vi "Main VERSION 1.0.vi"() -> ()   [LabVIEW 2017]
uses:
  <vilib>/addons/_Advanced Signal Processing/NI_AdvSigProcWA.lvlib
  <vilib>/addons/_Advanced Signal Processing/NI_AdvSigProcTSA.lvlib
  <vilib>/addons/Control Design/_Model Construction/NI_LinSys_Model Creation.lvlib
  <vilib>/addons/Control Design/_Model Conversions/NI_CD_Continuous and Discrete.lvlib
  <vilib>/addons/Control Design/_Model Construction/Data Typedefs.llb/CD DtoC Conversion Method.ctl
  <vilib>/addons/Control Design/_Model Construction/NI_LinSys_Data Typedefs.lvlib
  <vilib>/Analysis/NI_AALBase.lvlib
  Data.ctl
  <vilib>/Math Plots/3D Math Plots/3D Surface/3D Surface Datatype/3D Surface Datatype.lvclass
  <vilib>/addons/Control Design/_Dynamic Analysis/NI_CD_Dynamic Analysis.lvlib
  <vilib>/platform/TimedLoop/XDataNode/XDataNode.xnode
  <vilib>/Platform/TimedLoop/XDataNode/nitl_modes.ctl
  <vilib>/Platform/TimedLoop/XDataNode/XDNodeRunTimeDep.lvlib
  <vilib>/Platform/TimedLoop/XDataNode/wakeup.ctl
  <vilib>/Platform/TimedLoop/XDataNode/timing_clust.ctl
  <vilib>/addons/Control Design/_Model Construction/Model Creation.llb/Model Creation SubVI/cd_Create Transfer Function Model.vi
  <vilib>/addons/Control Design/_Model Conversions/NI_CD_Model Type.lvlib
  <vilib>/Analysis/NI_AALPro.lvlib
  <vilib>/addons/Control Design/_Time Response Analysis/NI_CD_Time Response.lvlib
  <vilib>/Utility/file.llb/Read Delimited Spreadsheet (DBL).vi
  <vilib>/ptbypt/NI_PtbyPt.lvlib
  <vilib>/Utility/file.llb/Write Delimited Spreadsheet (DBL).vi
  <vilib>/addons/Control Design/_Dynamic Analysis/Dynamic Analysis.llb/Dynamic Analysis subVI/cd_Damping Ratio and Natural Frequency (State-Space).vi
  <vilib>/addons/Control Design/_Time Response Analysis/Time Response.llb/Time Response subVI/cd_Linear Simulation (Transfer Function).vi
  <vilib>/addons/Control Design/_Model Conversions/Continuous and Discrete.llb/Continuous and Discrete SubVI/cd_Convert Discrete to Continuous (TF).vi
  <vilib>/addons/Time Series Analysis/Modeling and Prediction.llb/TSA ARMA Modeling (Waveform).vi
  <vilib>/addons/Control Design/_Dynamic Analysis/Dynamic Analysis.llb/Dynamic Analysis subVI/cd_Damping Ratio and Natural Frequency (Transfer Function).vi
  <vilib>/addons/Control Design/_Model Conversions/Model Type.llb/Model Conversion SubVI/cd_Convert Transfer Function to State-Space Model.vi
  <vilib>/Analysis/3filter.llb/IIR Filter (DBL).vi
  <vilib>/addons/Wavelet Analysis/application.llb/WA Detrend (Waveform).vi
  <vilib>/addons/Time Series Analysis/Correlation and Spectral Analysis.llb/TSA ARMA Spectrum (Waveform).vi
  <vilib>/Math Plots/3D Math Plots/3D Surface/3D Surface Datatype/Public/Plot Helper (Vector).vi
  State.ctl
  <vilib>/Math Plots/3D Math Plots/3D Surface/3D Surface XCtrl/3D Surface.xctl
panel:
  out "Poles":cdb[](array[numeric]) format="%.2f"
  out "Damping Ratios":dbl[](array[numeric]) format="%.2f"
  out "Natural Frequencies":dbl[](array[numeric]) format="%.2f"
  out "subarray 2":dbl[](array[numeric])
  out "AR coeff test 2":dbl[](array[numeric])=[1.0, -3.469, 4.669, -2.879, 0.6897]
  out "subarray":dbl[][](array[numeric])
  in  "Tab Control 2":enum32{"Data", "Preprocessed data"}(tab)
  out "Real-time data":waveform(dbl)(graph)={"t0"=timestamp(3467964116.0127993 s since 1904-01-01), "dt"=0.02, "Y"=array[30000 elements]}
  out "Preprocessed data":waveform(dbl)(graph)={"t0"=timestamp(3467964116.0127993 s since 1904-01-01), "dt"=0.2, "Y"=array[3000 elements]}
  in  "Tab Control":T1(tab)=enum."Options"
  out "Critical Damping [%]":dbl=11.530156484123282
  out "Critical Frequency [Hz]":dbl=1.626086044993813
  out "Estimated complex plane":cluster{dbl[], dbl[]}(graph)={[-1.1780360817698377, -0.5023745738423925, -1.9397187258807729], [10.148858009104277, 3.227170083530164, 12.249765461704891]}
  out "Damping ratio evolution":dbl[][](graph)=[[11.530156484123282, 8.701215529283058, 2.189395909955882, 2.4614029943222535, 5.193514233637378, 4.3692184421257805, 4.91283055168465, 4.380817107946644, 2.1306948942275286, 8.227924724815844, 2.674410475393449, 9.21941081019913]]
  in  "Number of critical modes":i32=1
  in  "Length of Spectra [s]":dbl=12.0
  out "Spectrogram":refnum<class "3D Plot Datatype.lvclass">[](xcontrol)
  in  "dB Scale":bool=TRUE
  out "Spectrum":cluster{"f0":dbl, "df":dbl, "S(f)":dbl[]}(graph)={"f0"=0.0, "df"=0.0048828125, "S(f)"=[53.04783210228587, 56.63653445699592, 58.023891931913106, 59.67116404097662, 61.284054847341054, 62.76981524500722, 64.11687043737376, 65.33794997742491, 66.45015373901528, 67.46886875000477, 68.40631100060692, 69.27151565501251, 70.07073014946974, 70.80788585589455, 71.48506608411563, 72.10296533438401, 72.66135194305483, 73.15953947791074, 73.59685537036363, 73.97307660858725, 74.28878941943108, 74.54562919953614, 74.74637114057295, 74.89486760408374, 74.99585665068564, 75.05468730953243, 75.0770149019896, 75.06851380977426, 75.03464026528596, 74.98046048345269, 74.91054484865359, 74.82891934483663, 74.73906102646188, 74.64392380160663, 74.54598253767928, 74.44728617051356, 74.34951322777977, 74.25402551961022, 74.1619175504306, 74.0740604811893, 73.99114030974818, 73.9136904467079, 73.84211914252114, 73.7767323478459, 73.71775262048499, 73.66533466900506, 73.61957807164293, 73.5805376459866, 73.54823188003344, 73.52264977404724, 73.50375638784266, 73.49149734072392, 73.4858024713342, 73.48658883165905, 73.49376316265318, 73.50722397761325, 73.52686336266768, 73.55256859076123, 73.58422363541801, 73.62171066243388, 73.66491157037783, 73.71370964298946, 73.76799136641728, 73.82764844926844, 73.89258006024016, 73.96269526207116, 74.03791556557854, 74.1181774458125, 74.20343454441851, 74.29365911777792, 74.38884207004048, 74.48899062945569, 74.59412239354747, 74.70425411613539, 74.81938331104598, 74.93946063995493, 75.06435135111367, 75.19378503485144, 75.32729498078686, 75.46415167436817, 75.6032993266386, 75.74330901487231, 75.88236539108851, 76.01830367318581, 76.14870760287604, 76.27106668197574, 76.38297473443528, 76.48233722171956, 76.567548282804, 76.63760408035796, 76.69213526024357, 76.73136176637777, 76.75599006111887, 76.76708083903773, 76.76591406961832, 76.75387077046256, 76.73234153456316, 76.70266377607953, 76.6660844104162, 76.62374225963825, 76.57666412087157, 76.5257692499374, 76.47187827374617, 76.41572380516381, 76.35796107933896, 76.29917770086449, 76.23990210798334, 76.18061067647423, 76.1217335591145, 76.06365943561697, 76.00673936964108, 75.95128995956487, 75.89759594482322, 75.8459123998421, 75.79646661853478, 75.74945976672043, 75.70506835869804, 75.66344559760455, 75.62472260666664, 75.58900956937647, 75.55639679030908, 75.52695568412523, 75.50073969773588, 75.4777851692011, 75.45811212635587, 75.4417250281344, 75.42861345190909, 75.41875273072952, 75.41210454504176, 75.40861747421977, 75.40822751400344, 75.41085856667677, 75.41642291151614, 75.42482166367071, 75.43594523019257, 75.44967377239409, 75.46587768405924, 75.48441809525055, 75.50514741151336, 75.52790989815483, 75.55254231893963, 75.57887463796702, 75.606730792646, 75.63592954453935, 75.66628541338444, 75.69760969780361, 75.72971158409061, 75.76239934201378, 75.795481603843, 75.82876871983562, 75.8620741802788, 75.8952160909746, 75.92801868588295, 75.96031385763509, 75.99194268394, 76.02275692567179, 76.05262047079196, 76.0814106973545, 76.10901972876889, 76.13535555532907, 76.16034299778357, 76.18392449140839, 76.20606067257935, 76.22673075411002, 76.2459326804616, 76.26368305914585, 76.28001687001027, 76.29498695938368, 76.30866333104413, 76.32113225044141, 76.33249518238651, 76.34286758537615, 76.35237758776404, 76.36116457208469, 76.36937769399348, 76.37717436156206, 76.38471869915384, 76.3921800179218, 76.399731312252, 76.40754779837235, 76.41580550799458, 76.4246799463977, 76.43434482091358, 76.44497084244557, 76.45672459952794, 76.46976750158741, 76.48425478555691, 76.50033457786182, 76.51814700209086, 76.537823321419, 76.55948510411083, 76.58324340025439, 76.60919791832202, 76.6374361913053, 76.66803272411654, 76.70104811679032, 76.73652816184644, 76.77450291907336, 76.81498577698629, 76.85797251727257, 76.90344040650483, 76.95134734798053, 77.00163113524022, 77.0542088569138, 77.10897650910722, 77.16580887543216, 77.22455973475066, 77.28506245152305, 77.34713099231259, 77.41056139398341, 77.475133684643, 77.54061422858938, 77.6067584336654, 77.67331372673053, 77.74002267438226, 77.80662610573624, 77.87286608565972, 77.93848859279498, 78.00324577763865, 78.06689771036126, 78.12921357240282, 78.18997229504036, 78.24896269622393, 78.30598320836378, 78.36084131989398, 78.41335286956605, 78.46334133381099, 78.51063723532924, 78.55507777800551, 78.59650678285838, 78.63477496585358, 78.66974056458548, 78.70127028997815, 78.72924055336367, 78.75353889979947, 78.77406556576946, 78.79073507334817, 78.80347777292985, 78.8122412518888, 78.81699153604242, 78.81771402347431, 78.81441410508471, 78.807117442166, 78.79586988743347, 78.78073705146184, 78.76180353070973, 78.7391718257197, 78.7129609882886, 78.68330504420013, 78.65035124345292, 78.61425819290841, 78.57519392716361, 78.53333397258037, 78.48885945721293, 78.44195531637583, 78.39280864032669, 78.34160720757664, 78.28853824527842, 78.23378745760364, 78.1775383646809, 78.11997199928643, 78.06126701696634, 78.00160028874863, 77.94114806552857, 77.88008783149982, 77.81860100322533, 77.75687668454131, 77.69511676008476, 77.63354270795473, 77.57240464286238, 77.51199327525148, 77.45265570160778, 77.39481624025024, 77.33900390797915, 77.28588860152158, 77.23632858870927, 77.19143246487005, 77.15263912661203, 77.12181919737093, 77.10139998238675, 77.09451208662946, 77.10514698357909, 77.1382975261337, 77.20002317838411, 77.29733540865345, 77.43774052768978, 77.62823161225614, 77.87354824854364, 78.17371984562733, 78.52135621237176, 78.89977446830142, 79.2834689612792, 79.64200391820367, 79.94678678707898, 80.17810549628706, 80.32909021423254, 80.40498736340558, 80.41896645675713, 80.38714023757896, 80.32483671152525, 80.2447019035565, 80.15623070884602, 80.06607714178779, 79.97864663238913, 79.89669770700486, 79.8218432814422, 79.75492917142036, 79.69630395356339, 79.64600440896002, 79.6038796954954, 79.56967279153454, 79.54307288267267, 79.52374832109005, 79.51136675797247, 79.50560689714834, 79.50616483455582, 79.51275694395522, 79.52512059701962, 79.5430135589285, 79.56621260467892, 79.59451170608011, 79.62772001095674, 79.66565975190154, 79.70816416702898, 79.75507547967509, 79.80624296130985, 79.86152108773445, 79.92076779005671, 79.98384279707365, 80.05060606328794, 80.1209162760194, 80.19462943540331, 80.27159750214368, 80.35166710948391, 80.43467833782597, 80.52046355267608, 80.60884630905795, 80.69964032816455, 80.79264855477103, 80.88766230675424, 80.98446053089533, 81.08280918189732, 81.18246074412212, 81.28315391780771, 81.38461349329644, 81.48655043790035, 81.58866222022453, 81.69063339583282, 81.7921364758338, 81.8928330960746, 81.99237549899337, 82.09040833272722, 82.18657076287359, 82.28049888163618, 82.37182838750634, 82.46019749706196, 82.54525004031949, 82.6266386843919, 82.70402822988488, 82.77709893456618, 82.84554984510027, 82.90910216821055, 82.96750279929881, 83.0205282664879, 83.06798956633493, 83.10973870024924, 83.14567821839111, 83.17577580604392, 83.20008697857843, 83.21879033153864, 83.23224144991188, 83.24105310440208, 83.24620954319899, 83.24921870324471, 83.25229252868525, 83.25851394982814, 83.27189246791492, 83.29713858822798, 83.33895686091842, 83.40078581729284, 83.48329369452597, 83.5834075564926, 83.6946918626584, 83.80914630314666, 83.9194939800654, 84.02078048103141, 84.11077450135917, 84.18945935657379, 84.25819390539944, 84.31896225289465, 84.37386809960977, 84.42486082458214, 84.47362219262848, 84.52154491008937, 84.56975518463469, 84.6191513946612, 84.67044469704172, 84.72419543129335, 84.7808433678376, 84.84073180065857, 84.90412625530703, 84.9712287814767, 85.0421887491838, 85.11711092933817, 85.1960614866747, 85.27907237543178, 85.366144514999, 85.4572500341974, 85.55233380573867, 85.65131444275491, 85.75408489337823, 85.86051274404058, 85.97044032496017, 86.08368470022344, 86.2000376184273, 86.31926549679474, 86.44110951099279, 86.56528586366412, 86.69148630607677, 86.81937898845217, 86.94860971456819, 87.07880367424393, 87.20956772236228, 87.3404932642739, 87.47115979393969, 87.60113911239554, 87.73000022976, 87.85731492419461, 87.98266389667822, 88.10564342253977, 88.22587236147383, 88.3429993499442, 88.4567099666591, 88.56673363657677, 88.67285002492687, 88.77489467267074, 88.8727636403219, 88.96641695838639, 89.05588072856739, 89.1412477774557, 89.22267682950323, 89.30039023358225, 89.37467034199577, 89.44585469740042, 89.51433022763241, 89.58052667814718, 89.6449095255229, 89.70797261362961, 89.77023073836328, 89.83221238000688, 89.8944527475736, 89.95748726030781, 90.02184555101928, 90.08804603676572, 90.15659106659064, 90.22796262489769, 90.30261854328616, 90.380989153439, 90.46347429869138, 90.55044061170233, 90.64221895956518, 90.73910195507645, 90.84134143317605, 90.94914579438051, 91.062677122183, 91.18204798899406, 91.30731787566103, 91.43848914369735, 91.57550251820746, 91.71823206462797, 91.8664796756997, 92.01996912871296, 92.17833982935551, 92.34114042963648, 92.50782259498837, 92.67773530013969, 92.85012015289084, 93.02410837428519, 93.19872019281603, 93.37286752304267, 93.54536087204167, 93.71492142038328, 93.88019912304051, 94.03979743538294, 94.19230486438343, 94.33633296933988, 94.47055971554589, 94.5937762851988, 94.70493468147838, 94.80319286424029, 94.88795387440493, 94.9588955525746, 95.01598807987202, 95.05949761483718, 95.0899756234817, 95.1082348876195, 95.1153144006739, 95.1124362317316, 95.10095785179813, 95.08232336383243, 95.05801663917848, 95.02951866998893, 94.99827064726611, 94.96564349614025, 94.93291393519425, 94.90124662329674, 94.87168162629092, 94.84512626132259, 94.82235032847149, 94.80398378321688, 94.79051600716397, 94.78229597263946, 91.76923279427284]}
  out "AR Coeff":dbl[](array[numeric])=[1.0, 0.2597816046489246, 0.2169384834121149, -0.679920142435816, -0.14595364680322792, 0.05002853302205009, 0.4579510483015735, 0.33236397122107786, -0.23625030751664058, -0.18717706840003662, -0.2062523669387352, 0.006685880060599296, 0.07110018702253204, 0.058723568346406144, 0.029083213351701387, 0.04124721740773827, 0.05689913231139613, 0.03808009033984788, 0.03677353221719321, 0.025432779832026717, 0.047521341239954946, 0.030318507891188288, 0.0798326201716732, 0.020455322957894737, 0.031484626629290524, -0.006461565839629831]
  out "MA Coeff":dbl[](array[numeric])=[1.0, -0.6848360549660951, 0.6884899387060236, -1.383587023284228, 0.9145041211231907, -0.7466132797884354, 0.988179180636961, -0.5622742582232239, 0.09840748978464724, -0.26486368933416604, -0.03646716818404465]
  out "Picture 9":picture
  out "Picture 8":picture
  out "Picture 7":picture
  out "Picture 6":picture
  out "Picture 5":picture
  out "Picture 4":picture
  out "Picture 3":picture
  out "Picture 2":picture
  out "Picture 1":picture
  out "Std of Damping":dbl[](array[numeric])=[3.167813045881809]
  out "Mean Damping [%]":dbl[](array[numeric])=[5.49924934647624]
  out "Frequency[Hz]":dbl[](array[numeric])=[1.626086044993813, 0.5198061588603065, 1.9739015777045272] format="%.4f"
  out "Damping Ratio [%]":dbl[](array[numeric])=[11.530156484123282, 15.381771713903165, 15.639879258359347] format="%.4f"
  out "Complex Poles":cdb[](array[numeric])=[-1.1780360817698377+10.148858009104277i, -0.5023745738423925+3.227170083530164i, -1.9397187258807729+12.249765461704891i] format="%.4f"
  out "Format":string="a0*z^4+a1*z^3+a2*z^2+a3*z^1+a4"
  out "Format":string="b0*z^3+b1*z^2+b2*z^1+b3"
  in  "MA coeff test":dbl[](array[numeric])=[1.0, -2.175, 1.45, 5.0]
  in  "AR coeff test":dbl[](array[numeric])=[1.0, -3.469, 4.669, -2.879, 0.6897]
  in  "Simulation/PRL":bool=TRUE
  in  "Upper Damping [%]":dbl=20.0
  in  "Lower Damping [%]":dbl
  in  "Upper Frequency [Hz]":dbl=2.0
  in  "Lower Frequency [Hz]":dbl=0.08
  in  "Signal Selection":enum32{"Mag", "Phase", "Analog"}(radio)=enum."Analog"
  in  "Downsampling Ratio":dbl=10.0
  in  "Low-pass Filter [Hz]":dbl=2.5
  in  "Low-pass Filter Order":u32=5
  in  "Detrend Cut-off Frequency":dbl=0.05
  in  "MA Order":i32=10
  in  "Sampling Frequency":dbl=50.0
  in  "AR Order":i32=25
  in  "Parcel Length (Simulation)":i32=30000
  in  "Refresh Rate [s]":i32=10
  in  "Std Threshold":dbl=1.35
  out "Parcel Length (SDK or Simulation)":i32=30000
  out "Simulation":bool=TRUE
  in  "stop":bool
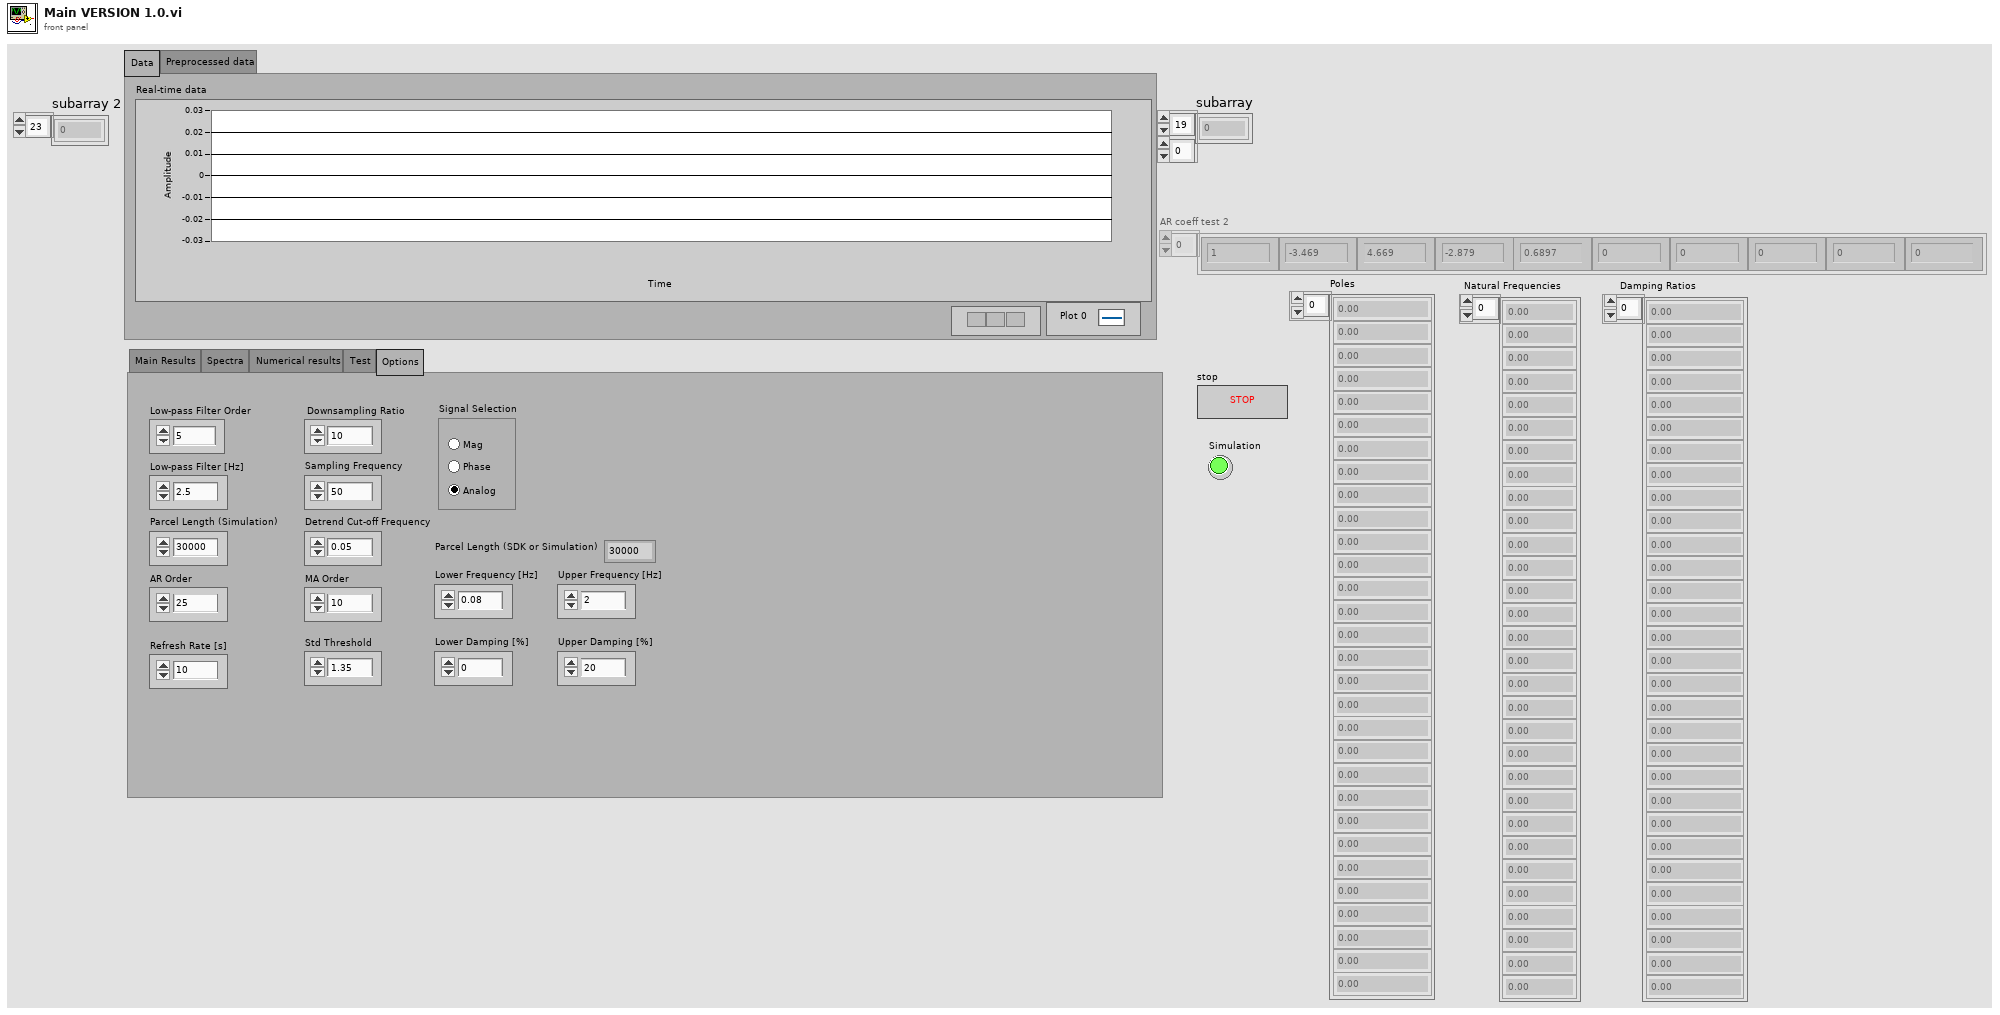
[diagram p1: front panel]
types:
  T1 = enum32{"Main Results", "Spectra", "Numerical results", "Test", "Options"}
  T2 = typedef "State.ctl" = enum16{"Initialize", "Read Real Data", "Read Simulated Data", "Preprocessing", "Compute AR/MA Coeffs", "Get Spectrum"}
  T3 = typedef "Data.ctl" = cluster{"Waveform":waveform(dbl), "Parcel Length":i32, "AR Order":i32, "Sampling Frequency":dbl, "MA Order ":i32}
  T4 = typedef "XDNodeRunTimeDep.lvlib/timing_clust.ctl" = cluster{"Expected End [f-1]":u64, "Actual End [f-1]":u64, "Finished Late? [f-1]":bool, "Expected End [i-1]":u64, "Actual End [i-1]":u64, "Finished Late? [i-1]":bool, "Expected Start [i]":u64, "Actual Start [i]":u64, "Expected Start [f]":u64, "Actual Start [f]":u64, "Source Name":string, "Structure Name":string, "Period":i64, "Deadline":i64, "Offset":i64, "Start":i64, "Priority":i32, "Timeout":i32, "Mode":T5, "Wakeup Reason":T6, "Error":errorcluster, "Source Type":string, "Secondary Source Type":string, "Global End Time":u64, "Global Start Time":u64, "Frame Duration":u64, "Iteration Duration":u64, "Assigned CPU":i32, "I/O Scan Engine Mode":u32}
  T5 = typedef "XDNodeRunTimeDep.lvlib/nitl_modes.ctl" = enum32{"No Change", "Process missed periods, maintain original phase", "Discard missed periods, maintain original phase", "Process missed periods, ignore original phase", "Discard missed periods, ignore original phase"}
  T6 = typedef "XDNodeRunTimeDep.lvlib/wakeup.ctl" = enum32{"Normal", "Aborted", "Asynchronous wakeup", "Timing source error", "Timed loop error", "Timeout"}
  T7 = typedef "State.ctl" = enum16{"Initialize", "Read Real Data", "Read Simulated Data", "Preprocessing", "Compute AR Coeff", "Get Spectrum"}
  T8 = enum8{"Enabled", "Disabled", "Disabled and Grayed Out"}
  T9 = typedef "NI_LinSys_Model Typedefs.lvlib/CD Transfer Function Model (MIMO).ctl" = cluster{"properties":T10, "transfer function(s)":T11[][]}
  T10 = typedef "NI_LinSys_Model Typedefs.lvlib/CD General Elements.ctl" = cluster{"Model name":string, "Input names":string[], "Output names":string[], "Input Delays":dbl[], "Output Delays":dbl[], "Sampling Time":dbl, "Notes":string}
  T11 = typedef "NI_LinSys_Model Typedefs.lvlib/CD Transfer Function Model (SISO).ctl" = cluster{"Numerator":dbl[], "Denominator":dbl[], "delay":dbl}
  T12 = typedef "NI_LinSys_Data Typedefs.lvlib/CD MIMO Time Response Data.ctl" = cluster{"Time":dbl[], "Outputs Data":dbl[][][], "States Data":dbl[][][], "plot type":T13}
  T13 = typedef "NI_LinSys_Data Typedefs.lvlib/CD Plot Types Enum.ctl" = enum16{"bode-magnitude", "bode-phase", "nichols", "nyquist", "singular values", "step", "impulse", "initial", "simulation", "nyquist with separation"}
  T14 = typedef "NI_LinSys_Data Typedefs.lvlib/CD DtoC Conversion Method.ctl" = u16
  T15 = typedef "NI_LinSys_Model Typedefs.lvlib/CD State Space Model (MIMO).ctl" = cluster{"properties":T10, "A":dbl[][], "B":dbl[][], "C":dbl[][], "D":dbl[][], "StateNames":string[], "Transport Delay":dbl[][]}
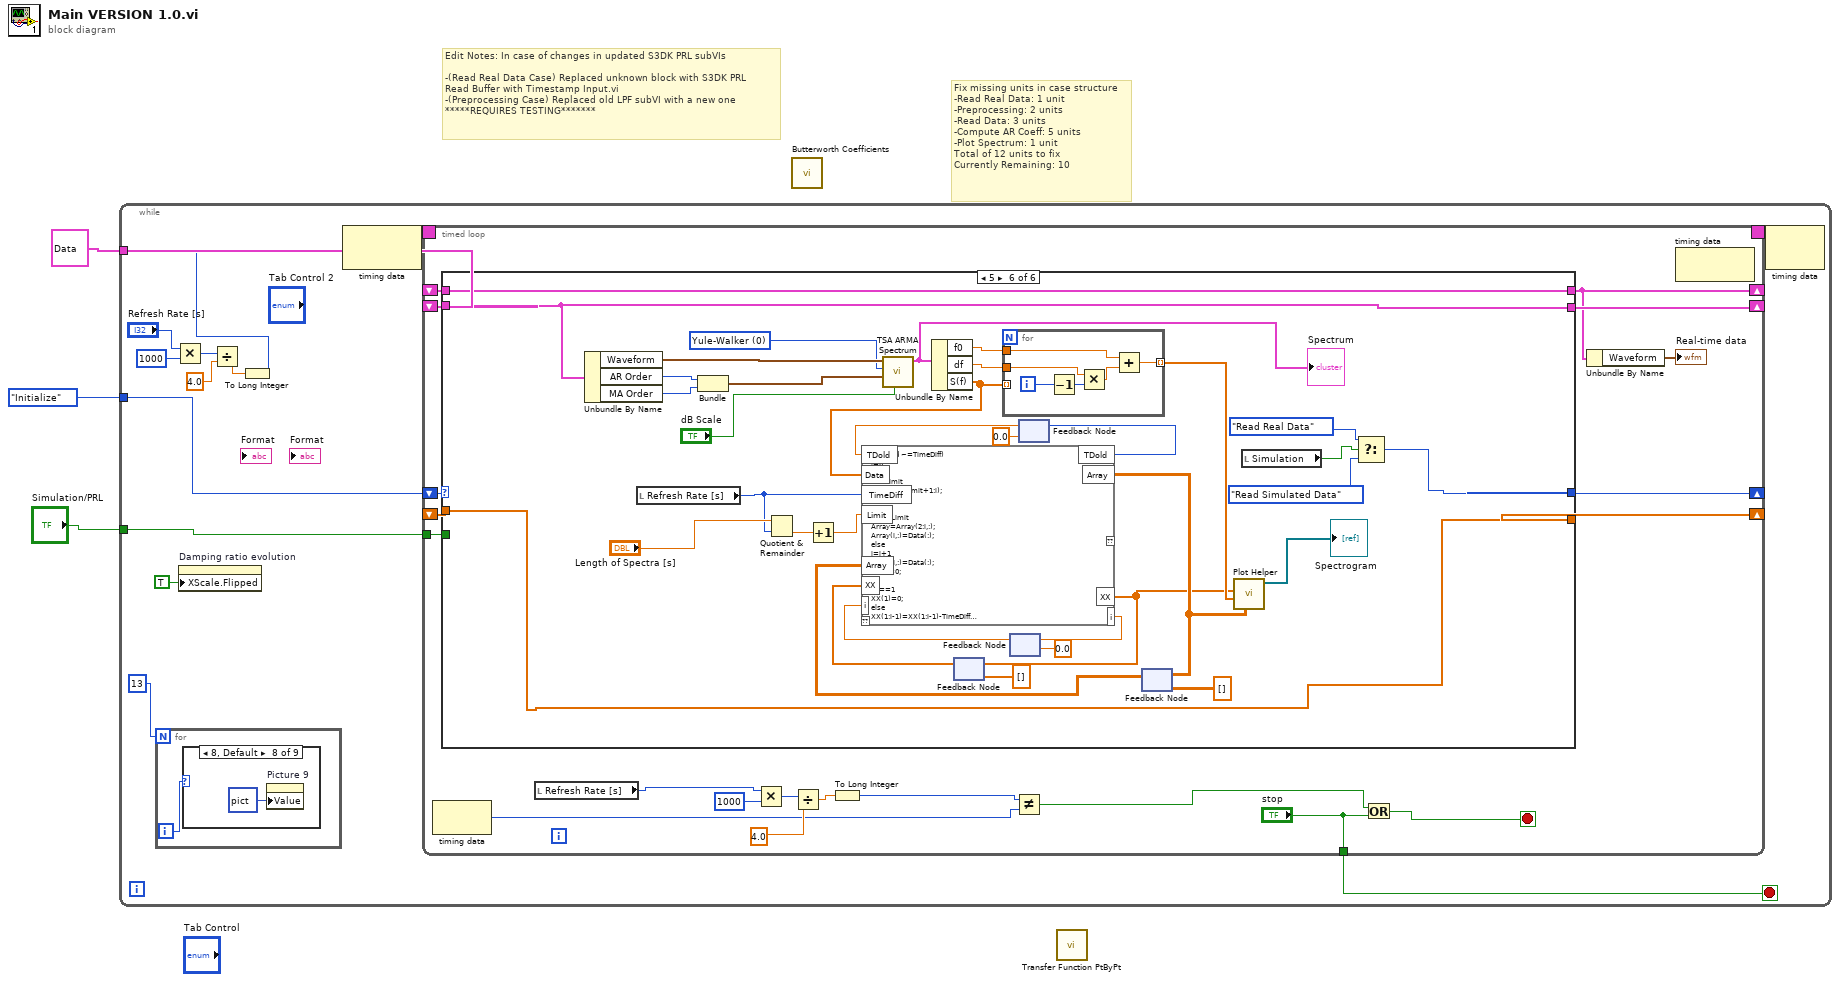
[diagram p0: block diagram]
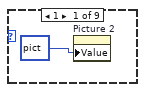
[diagram p2: hidden frame]
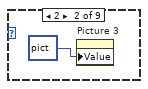
[diagram p3: hidden frame]
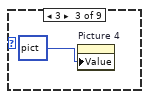
[diagram p4: hidden frame]
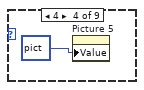
[diagram p5: hidden frame]
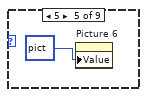
[diagram p6: hidden frame]
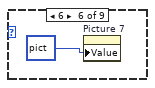
[diagram p7: hidden frame]
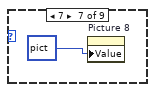
[diagram p8: hidden frame]
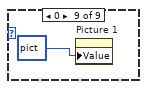
[diagram p9: hidden frame]
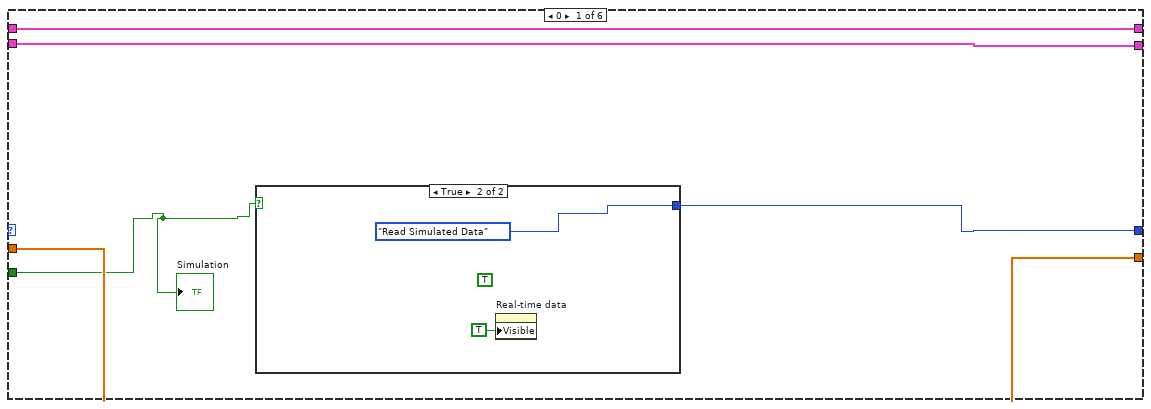
[diagram p10: hidden frame]
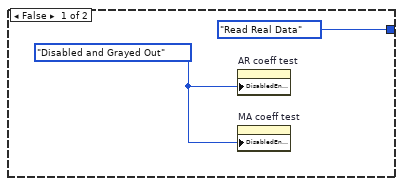
[diagram p11: hidden frame]
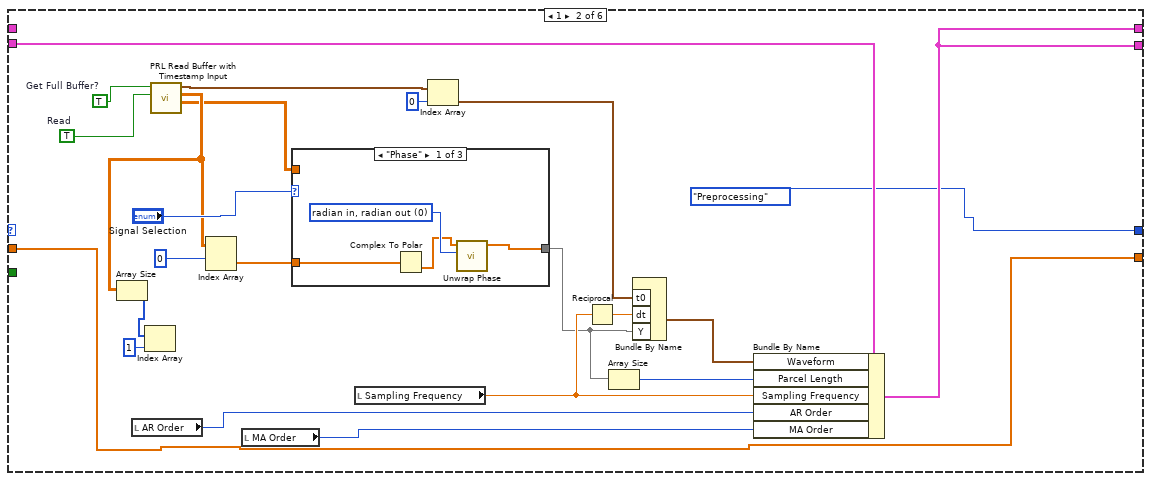
[diagram p12: hidden frame]
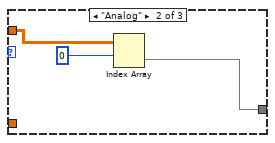
[diagram p13: hidden frame]
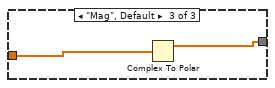
[diagram p14: hidden frame]
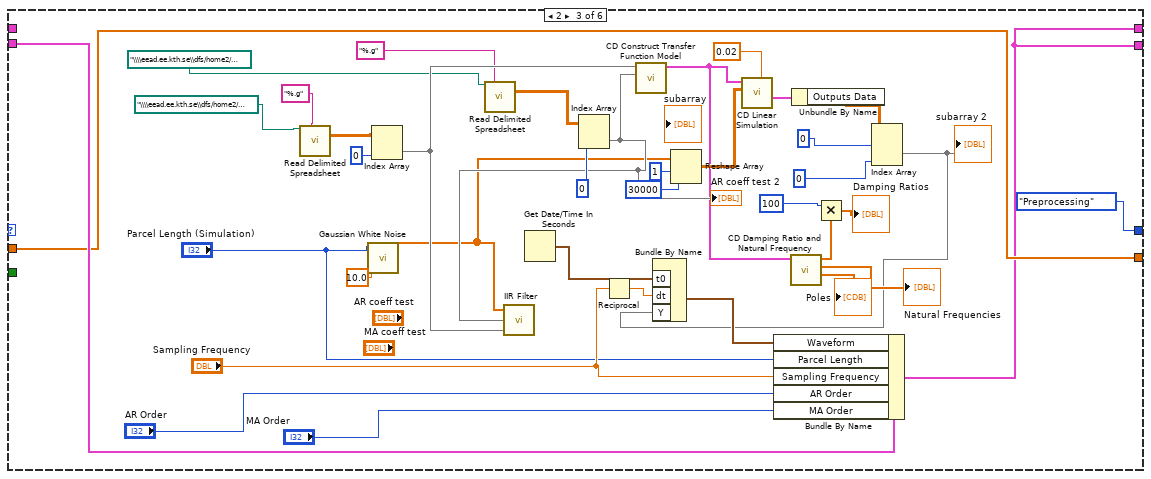
[diagram p15: hidden frame]
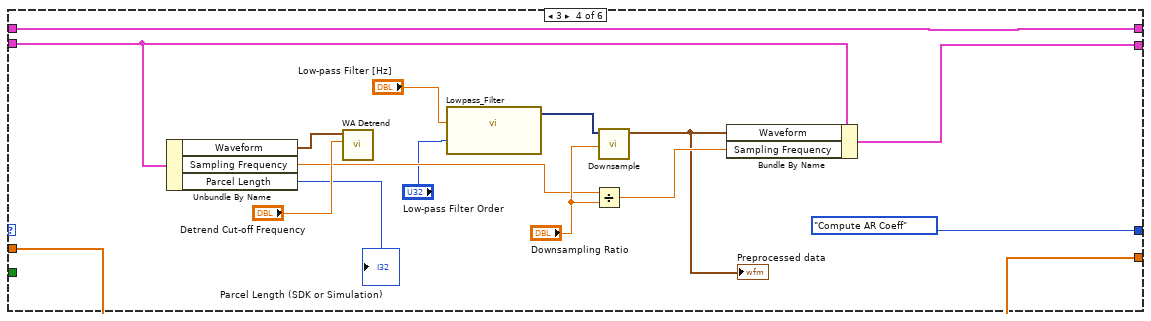
[diagram p16: hidden frame]
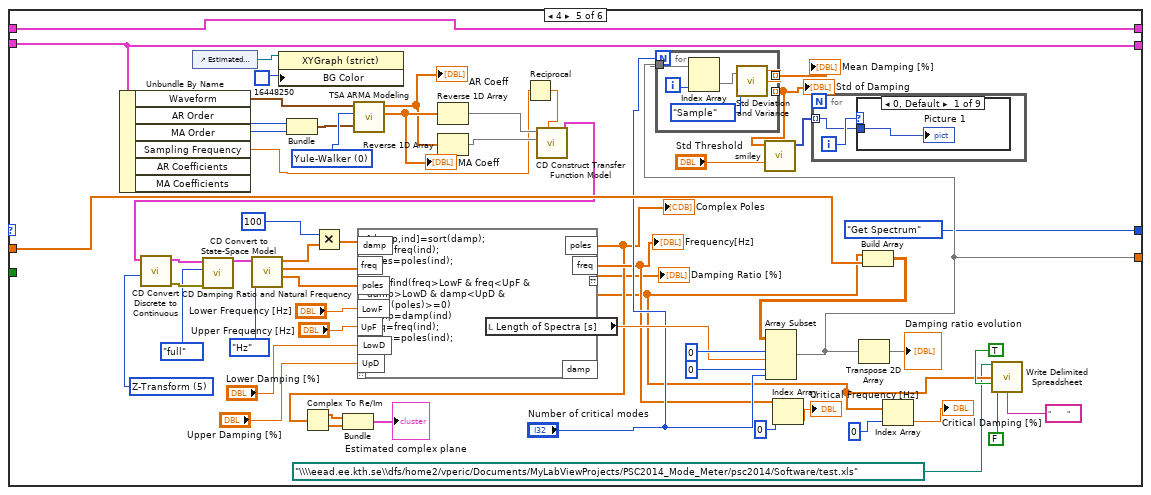
[diagram p17: hidden frame]
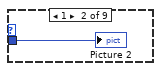
[diagram p18: hidden frame]
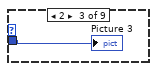
[diagram p19: hidden frame]
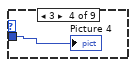
[diagram p20: hidden frame]
diagram:
  # "Edit Notes: In case of changes in updated S3DK PRL subVIs\n\n-(Read Real Data Case) Replaced unknown block with S3DK PRL\nRead Buffer with Timestamp Input.vi  \n-(Preprocessing Case) Replaced old LPF subVI with a new one\n*****REQUIRES TESTING*******"
  # "Fix missing units in case structure\n-Read Real Data: 1 unit\n-Preprocessing: 2 units\n-Read Data: 3 units\n-Compute AR Coeff: 5 units\n-Plot Spectrum: 1 unit\nTotal of 12 units to fix\nCurrently Remaining: 10"
  n1 = while {
    tunnel: State."Initialize" ("Enum") -> [w7]
    tunnel: T3 {"Waveform"={"t0"=timestamp(0 s since 1904-01-01), "dt"=1.0, "Y"=[]}, "Parcel Length"=0, "AR Order"=0, "Sampling Frequency"=0.0, "MA Order "=0} ("Cluster") -> [w15]
    tunnel: "Simulation/PRL" -> [w5]
    stop <- w8 stop-if-true
    n2 = for {
      N: 13 -> [_]
      i -> [w18]
      n3 = case shown="8, Default" w18 {
        frame 1 {
          n4 = property on="Picture 2" class="Pict"("Value"=picture bytes[260130] ("Picture 9")) -> ()  [unwired: 2 in, 2 out]
        }
        frame 2 {
          n5 = property on="Picture 3" class="Pict"("Value"=picture bytes[260130] ("Picture 9")) -> ()  [unwired: 2 in, 2 out]
        }
        frame 3 {
          n6 = property on="Picture 4" class="Pict"("Value"=picture bytes[260130] ("Picture 9")) -> ()  [unwired: 2 in, 2 out]
        }
        frame 4 {
          n7 = property on="Picture 5" class="Pict"("Value"=picture bytes[260130] ("Picture 9")) -> ()  [unwired: 2 in, 2 out]
        }
        frame 5 {
          n8 = property on="Picture 6" class="Pict"("Value"=picture bytes[260130] ("Picture 9")) -> ()  [unwired: 2 in, 2 out]
        }
        frame 6 {
          n9 = property on="Picture 7" class="Pict"("Value"=picture bytes[260130] ("Picture 9")) -> ()  [unwired: 2 in, 2 out]
        }
        frame 7 {
          n10 = property on="Picture 8" class="Pict"("Value"=picture bytes[260130] ("Picture 9")) -> ()  [unwired: 2 in, 2 out]
        }
        frame 8, Default {
          n11 = property on="Picture 9" class="Pict"("Value"=picture bytes[260130] ("Picture 9")) -> ()  [unwired: 2 in, 2 out]
        }
        frame 0 {
          n12 = property on="Picture 1" class="Pict"("Value"=picture bytes[260130] ("Picture 9")) -> ()  [unwired: 2 in, 2 out]
        }
      }
    }
    n13 = Multiply(x="Refresh Rate [s]", y=1000) -> (x*y=w12:i32)
    n14 = property on="Damping ratio evolution" class="WFGraph (strict)"("XScale.Flipped"=TRUE ("X Scale.Flipped")) -> ()  [unwired: 2 in, 2 out]
    n15 = Divide(x=w12, y=4.0) -> (x/y=w10:dbl)
    n16 = To Long Integer(number=w10) -> (32bit integer=w9:i32)
    n17 = node-c288(w9) -> (w17:T4)
    n18 = timed-loop {
      shift-right: [w32] -> _
      shift-left: w15 -> [w46]
      shift-right: [w45] -> _
      shift-left: w7 -> [w47]
      timing: w17 -> [_]
      timing-out: [_] -> w16
      tunnel: ["stop"] -> w8
      shift-right: [w35] -> _
      shift-left: _ -> [w34]
      tunnel: w5 -> [w33]
      shift-right: [w30] -> _
      shift-left: _ -> [w29]
      stop <- w44 stop-if-true
      n19 = node-c288() -> (w28:i64)  [unwired: 1 in]
      n20 = case shown="5" w47 {
        tunnel: w46 -> [w54 w77 w129 w137 w201 w237]
        tunnel: [w54 w68 w121 w144 w201 w237] -> w32
        tunnel: [w55 State."Preprocessing" ("Enum") State."Preprocessing" ("Enum") State."Compute AR Coeff" ("Enum") State."Get Spectrum" ("Enum") w235] -> w45
        tunnel: [w53 w70 w122 w138 w176 w231] -> w35
        tunnel: w34 -> [w53 w70 w122 w138 w189 w231]
        tunnel: w33 -> [w52 _ _ _ _ _]
        tunnel: [w51 w68 w121 w136 w180 w226] -> w30
        tunnel: w29 -> [w51 _ _ w136 w180 w226]
        frame 0 {
          n21 = case shown="True" w52 {
            tunnel: [State."Read Real Data" ("Enum") State."Read Simulated Data" ("Enum")] -> w55
            frame False {
              w57 = T8."Disabled and Grayed Out" ("Disabled")
              n22 = property on="AR coeff test" class="Arr (strict)"("DisabledEnum"=w57) -> ()  [unwired: 2 in, 2 out]
              n23 = property on="MA coeff test" class="Arr (strict)"("DisabledEnum"=w57) -> ()  [unwired: 2 in, 2 out]
            }
            frame True {
              (unwired) TRUE ("Visible")
              n24 = property on="Real-time data" class="WFChart (strict)"("Visible"=TRUE) -> ()  [unwired: 2 in, 2 out]
            }
          }
          "Simulation" <- w52
        }
        frame 1 {
          w64 = TRUE  # Read
          w65 = TRUE  # Get Full Buffer?
          n25 = local read "AR Order"() -> (w80:i32)
          n26 = call <vilib>:"PRL Read Buffer with Timestamp Input.vi"("Get All Signals"=w64, "Get Full Buffer"=w65) -> ("Analog Signals"=w61:sgl[][], "Phasor Signals"=w62:csg[][], "Timestamp"=w63:timestamp[])  [unwired: 3 in, 4 out]
          n27 = Array Size(array=w62) -> (size(s)=w71:i32[])
          n28 = Index Array(array=w71, index=1) -> ()  [unwired: 1 out]
          n29 = Index Array "Index Array"(array=w62, index (row)=0) -> (element=w73:csg[])  [unwired: 1 in]
          n30 = local read "MA Order"() -> (w78:i32)
          n31 = case shown="\"Phase\"" "Signal Selection" {
            tunnel: [w83 w87 w91] -> w66
            tunnel: w73 -> [w86 _ w90]
            tunnel: w61 -> [_ w88 _]
            frame "Phase" {
              w85 = 0 items=["radian in, radian out", "radian in, degree out", "degree in, degree out", "degree in, radian out"] ("phase unit")
              n32 = Complex To Polar(r * e^(i*theta)=w86) -> (theta=w84:sgl[])  [unwired: 1 out]
              n33 = call <vilib>:"Unwrap Phase.vi"("phase unit"=w85, "Phase"=w84) -> ("Unwrapped Phase"=w83:dbl[])  [unwired: 8 in, 1 out]
            }
            frame "Analog" {
              n34 = Index Array(array=w88, index (row)=0) -> (element=w87:sgl[])  [unwired: 1 in]
            }
            frame "Mag", Default {
              n35 = Complex To Polar(r * e^(i*theta)=w90) -> (r=w91:sgl[])  [unwired: 1 out]
            }
          }
          n36 = local read "Sampling Frequency"() -> (w79:dbl)
          n37 = Index Array(array=w63, index=0) -> (element=w75:timestamp)
          n38 = Reciprocal(x=w79) -> (1/x=w82:dbl)
          n39 = Array Size(array=w66) -> (size(s)=w67:i32)
          n40 = Bundle By Name("t0"=w75, "dt"=w82, "Y"=w66) -> (w81:waveform(dbl))  [unwired: 1 in]
          n41 = Bundle By Name(cluster=w77, "Waveform"=w81, "Parcel Length"=w67, "Sampling Frequency"=w79, "AR Order"=w80, "MA Order"=w78) -> (w68:T3)
        }
        frame 2 {
          n42 = call-poly <vilib>:"Read Delimited Spreadsheet.vi"("file path (dialog if empty)"=path "\\\\eead.ee.kth.se\\dfs/home2/vperic/Documents/MyLabViewProjects/PSC2014_Mode_Meter/psc2014/Software/num.txt", "format (%.3f)"="%.g") -> ("all rows"=w97:dbl[][])  [unwired: 8 in, 5 out]
          n43 = call <vilib>:"Gaussian White Noise.vi"("standard deviation"=10.0, "samples"="Parcel Length (Simulation)") -> ("Gaussian noise pattern"=w114:dbl[])  [unwired: 8 in, 1 out]
          n44 = Index Array(array=w97, index (col)=0 ("disabled index (col)")) -> (element=w116:dbl[])  [unwired: 1 in]
          n45 = call-poly <vilib>:"Read Delimited Spreadsheet.vi"("file path (dialog if empty)"=path "\\\\eead.ee.kth.se\\dfs/home2/vperic/Documents/MyLabViewProjects/PSC2014_Mode_Meter/psc2014/Software/den.txt", "format (%.3f)"="%.g") -> ("all rows"=w96:dbl[][])  [unwired: 8 in, 5 out]
          n46 = Get Date/Time In Seconds() -> (seconds since 1Jan1904=w120:timestamp)
          n47 = Index Array(array=w96, index (col)=0 ("disabled index (col)")) -> (element=w115:dbl[])  [unwired: 1 in]
          "AR coeff test 2" <- w115
          n48 = call-poly <vilib>:"IIR Filter.vi"("Forward Coefficients"=w116, "Reverse Coefficients"=w115, "X"=w114) -> ()  [unwired: 1 in, 2 out]
          n49 = Reciprocal(x="Sampling Frequency") -> (1/x=w125:dbl)
          n50 = call-poly <vilib>:"CD Construct Transfer Function Model.vi"("Denominator"=w115, "Numerator"=w116) -> ("Transfer Function Model"=w107:T9)  [unwired: 8 in, 1 out]
          n51 = Reshape Array(w114, 1 ("dimension size"), 30000 ("dimension size")) -> (w113:dbl[][])
          n52 = call-poly <vilib>:"CD Linear Simulation.vi"("Delta t"=0.02, "Inputs"=w113, "Transfer Function Model"=w107) -> ("Simulation Data"=w112:T12)  [unwired: 6 in, 2 out]
          n53 = call-poly <vilib>:"CD Damping Ratio and Natural Frequency.vi"("Transfer Function Model"=w107) -> ("Poles"=→"Poles":cdb[], "Natural Frequencies"=→"Natural Frequencies":dbl[], "Damping Ratios"=w103:dbl[])  [unwired: 7 in, 1 out]
          n54 = Unbundle By Name(w112) -> ("Outputs Data"=w109:dbl[][][])
          n55 = Multiply(x=100 ("length"), y=w103) -> (x*y=→"Damping Ratios":dbl[])
          n56 = Index Array(array=w109, index (dim 0)=0 ("index"), index (dim 2)=0 ("length")) -> (element=w93:dbl[])  [unwired: 1 in]
          "subarray 2" <- w93
          n57 = Bundle By Name("t0"=w120, "dt"=w125, "Y"=w93) -> (w126:waveform(dbl))  [unwired: 1 in]
          n58 = Bundle By Name(cluster=w129, "Waveform"=w126, "Parcel Length"="Parcel Length (Simulation)", "Sampling Frequency"="Sampling Frequency", "AR Order"="AR Order", "MA Order"="MA Order") -> (w121:T3)
        }
        frame 3 {
          n59 = Unbundle By Name(w137) -> ("Waveform"=w132:waveform(dbl), "Sampling Frequency"=w140:dbl, "Parcel Length"=→"Parcel Length (SDK or Simulation)":i32)
          n60 = call-poly <vilib>:"WA Detrend.vi"("threshold frequency"="Detrend Cut-off Frequency", "signal"=w132) -> ()  [unwired: 7 in, 3 out]
          n61 = call "Lowpass_Filter.vi"("Order"="Low-pass Filter Order", "Lower Cut-Off"="Low-pass Filter [Hz]") -> ("Filtered Signal"=w131:dynamicdata)  [unwired: 3 in, 1 out]
          n62 = Divide(x=w140, y="Downsampling Ratio") -> (x/y=w139:dbl)
          n63 = call "Downsample.vi"("Divide by"="Downsampling Ratio", "Waveform in"=w131) -> ("Waveform out"=w135:waveform(dbl))  [unwired: 9 in]
          "Preprocessed data" <- w135
          n64 = Bundle By Name(cluster=w137, "Waveform"=w135, "Sampling Frequency"=w139) -> (w144:T3)
        }
        frame 4 {
          w199 = T14 5 items=["Zero-Order-Hold", "Tustin (Bilinear)", "Prewarp", "Forward", "Backward", "Z-Transform"] ("Method")
          w202 = u16 0 items=["Yule-Walker", "High order AR", "Polynomial"] ("method")
          n65 = Unbundle By Name(w201) -> ("Waveform"=w200:waveform(dbl), "AR Order"=w198:i32, "MA Order"=w197:i32, "Sampling Frequency"=w164:dbl)  [unwired: 2 out]
          n66 = control-ref of="Estimated complex plane"() -> (w192:refnum<vi>)
          n67 = property class="XYGraph (strict)"(reference=w192, "BG Color"=u32 16448250 ("Color Box")) -> ()  [unwired: 1 in, 2 out]
          n68 = Bundle("AR Order"=w198, "MA Order"=w197) -> (w196:cluster{"AR Order":i32, "MA Order ":i32})  [unwired: 1 in]
          n69 = call-poly <vilib>:"TSA ARMA Modeling.vi"("ARMA order"=w196, "method"=w202, "Xt"=w200) -> ("MA coefficients"=w158:dbl[], "AR coefficients"=w157:dbl[])  [unwired: 5 in, 2 out]
          "AR Coeff" <- w157
          "MA Coeff" <- w158
          n70 = Reverse 1D Array(array=w158) -> (reversed array=w172:dbl[])
          n71 = Reverse 1D Array(array=w157) -> (reversed array=w171:dbl[])
          n72 = local read "Length of Spectra [s]"() -> (w183:dbl)
          n73 = Reciprocal(x=w164) -> (1/x=w163:dbl)
          n74 = call-poly <vilib>:"CD Construct Transfer Function Model.vi"("Sampling Time (s)"=w163, "Denominator"=w171, "Numerator"=w172) -> ("Transfer Function Model"=w173:T9)  [unwired: 7 in, 1 out]
          n75 = call-poly <vilib>:"CD Convert Discrete to Continuous.vi"("Method"=w199, "Discrete Transfer Function Model"=w173) -> ("error out"=w162:errorcluster, "Continuous Transfer Function Model"=w151:T9)  [unwired: 8 in]
          n76 = call-poly <vilib>:"CD Convert to State-Space Model.vi"("error in (no error)"=w162, "Realization Type"=enum16{"minimum", "full"}."full", "Transfer Function Model"=w151) -> ("State-Space Model"=w160:T15)  [unwired: 7 in, 1 out]
          n77 = call-poly <vilib>:"CD Damping Ratio and Natural Frequency.vi"("Frequency Unit"=enum16{"Hz", "rad/s"}."Hz", "State-Space Model"=w160) -> ("Poles"=w174:cdb[], "Natural Frequencies"=w165:dbl[], "Damping Ratios"=w184:dbl[])  [unwired: 6 in, 1 out]
          n78 = Multiply(x=100 ("Numeric"), y=w184) -> (x*y=w182:dbl[])
          n79 = mathscript code="[damp,ind]=sort(damp);\nfreq=freq(ind);\npoles=poles(ind);\n\nind=find(freq>LowF & freq<UpF & damp>LowD & damp<UpD &  imag(poles)>=0)\ndamp=damp(ind)\nfreq=freq(ind);\npoles=poles(ind);"("damp"=w182, "freq"=w165, "poles"=w174, "LowF"="Lower Frequency [Hz]", "UpF"="Upper Frequency [Hz]", "LowD"="Lower Damping [%]", "UpD"="Upper Damping [%]") -> ("poles"=w159:cdb[], "freq"=w169:dbl[], "damp"=w149:dbl[])  [unwired: 1 in, 1 out]
          "Complex Poles" <- w159
          "Frequency[Hz]" <- w169
          "Damping Ratio [%]" <- w149
          n80 = Complex To Re/Im(x + iy=w159) -> (x=w195:dbl[], y=w194:dbl[])
          n81 = Bundle(w195, w194) -> (→"Estimated complex plane":cluster{dbl[], dbl[]})  [unwired: 1 in]
          n82 = Index Array(array=w169, index=0) -> (element=→"Critical Frequency [Hz]":dbl)
          n83 = Build Array(w149, w189) -> (w186:dbl[][])
          n84 = Array Subset "Array Subset"(array=w186, index (row)=0 ("index"), length (row)=w183, index (col)=0 ("index"), length (col)="Number of critical modes") -> (w176:dbl[][])
          n85 = for {
            N: "Number of critical modes" -> [_]
            tunnel: w176 -> [w218]
            tunnel: [w216] -> w181 mode=indexing
            tunnel: [w215] -> w178 mode=indexing
            i -> [w214]
            n86 = Index Array(array=w218, index (col)=w214) -> (element=w217:dbl[])  [unwired: 1 in]
            n87 = call <vilib>:"Std Deviation and Variance.vi"("X"=w217, "Weighting (Sample)"=enum16{"Sample", "Population"}."Sample") -> ("mean"=w216:dbl, "standard deviation"=w215:dbl)  [unwired: 1 out]
          }
          "Std of Damping" <- w178
          "Mean Damping [%]" <- w181
          n88 = call "smiley.vi"("std threshold"="Std Threshold", "damp"=w178) -> ("Array"=w179:picture[])  [unwired: 9 in]
          n89 = for {
            tunnel: w179 -> [w203] mode=indexing
            i -> [w204]
            n90 = case shown="0, Default" w204 {
              tunnel: w203 -> [w205 w206 w207 w208 w209 w210 w211 w212 w213]
              frame 0, Default {
                "Picture 1" <- w205
              }
              frame 1 {
                "Picture 2" <- w206
              }
              frame 2 {
                "Picture 3" <- w207
              }
              frame 3 {
                "Picture 4" <- w208
              }
              frame 4 {
                "Picture 5" <- w209
              }
              frame 5 {
                "Picture 6" <- w210
              }
              frame 6 {
                "Picture 7" <- w211
              }
              frame 7 {
                "Picture 8" <- w212
              }
              frame 8 {
                "Picture 9" <- w213
              }
            }
          }
          n91 = Transpose 2D Array(2D array=w176) -> (transposed array=→"Damping ratio evolution":dbl[][])
          n92 = Index Array(array=w149, index=0 ("length")) -> (element=→"Critical Damping [%]":dbl)
          n93 = call-poly <vilib>:"Write Delimited Spreadsheet.vi"("file path (dialog if empty)"=path "\\\\eead.ee.kth.se\\dfs/home2/vperic/Documents/MyLabViewProjects/PSC2014_Mode_Meter/psc2014/Software/test.xls", "1D data"=w149, "append to file? (new file:F)"=TRUE, "transpose? (no:F)"=FALSE, "delimiter (\\t)"="        " ("delimiter (\\t)")) -> ()  [unwired: 9 in, 2 out]
        }
        frame 5 {
          w239 = u16 0 items=["Yule-Walker", "High order AR", "Polynomial"] ("method")
          n94 = Unbundle By Name(w237) -> ("Waveform"=w251:waveform(dbl), "AR Order"=w254:i32, "MA Order"=w253:i32)
          n95 = local read "Refresh Rate [s]"() -> (w224:i32)
          n96 = Bundle("AR Order"=w254, "MA Order"=w253) -> (w252:cluster{"AR Order":i32, "MA Order ":i32})  [unwired: 1 in]
          n97 = Quotient & Remainder(x="Length of Spectra [s]", y=w224) -> (floor(x/y)=w223:dbl)  [unwired: 1 out]
          n98 = Increment(x=w223) -> (x+1=w222:dbl)
          n99 = call-poly <vilib>:"TSA ARMA Spectrum.vi"("dB on? (T)"="dB Scale", "ARMA order"=w252, "method"=w239, "Xt"=w251) -> ("PSD"=w238:cluster{"f0":dbl, "df":dbl, "S(f)":dbl[]})  [unwired: 5 in, 2 out]
          "Spectrum" <- w238
          n100 = Unbundle By Name(w238) -> ("f0"=w247:dbl, "df"=w246:dbl, "S(f)"=w243:dbl[])
          n101 = feedback #1(dbl[] [] ("XX")) -> (w245:dbl[])
          n102 = for {
            tunnel: w243 -> [_] mode=indexing
            tunnel: w247 -> [w256]
            tunnel: w246 -> [w258]
            tunnel: [w255] -> w234 mode=indexing
            i -> [w260]
            n103 = Decrement(x=w260) -> (x-1=w259:i32)
            n104 = Multiply(x=w258, y=w259) -> (x*y=w257:dbl)
            n105 = Add(x=w256, y=w257) -> (x+y=w255:dbl)
          }
          n106 = feedback #2(0.0 ("i")) -> (w250:dbl)
          n107 = feedback #3(0.0 ("TDold")) -> (w228:dbl)
          n108 = feedback #4(dbl[][] [] ("Array")) -> (w241:dbl[][])
          n109 = mathscript code="if (TDold ~=TimeDiff)\ni=0\nend\nif i>Limit\nXX=XX(i-Limit+1:i);\ni=Limit;\nend\nif i==Limit\nArray=Array(2:i,:);\nArray(i,:)=Data(:);\nelse\ni=i+1\nArray(i,:)=Data(:);\nXX(i)=0;\n\nif i==1\nXX(1)=0;\nelse\nXX(1:i-1)=XX(1:i-1)-TimeDiff\nXX(i)=0\nend\nend\n\nTDold=TimeDiff;"("Data"=w243, "Array"=w241, "i"=w250, "Limit"=w222, "XX"=w245, "TimeDiff"=w224, "TDold"=w228) -> ("Array"=w233:dbl[][], "i"=w248:dbl, "XX"=w230:dbl[], "TDold"=w229:i32)  [unwired: 1 in, 1 out]
          n110 = feedback-in #1(w230) -> ()
          n111 = feedback-in #2(w248) -> ()
          n112 = feedback-in #3(w229) -> ()
          n113 = feedback-in #4(w233) -> ()
          n114 = call-poly <vilib>:"Plot Helper.vi"("z matrix"=w233, "y vector"=w234, "x vector"=w230) -> ("3D Plot lvclass Array out"=→"Spectrogram":refnum<class "3D Plot Datatype.lvclass">[])  [unwired: 3 in, 5 out]
          n115 = local read "Simulation"() -> (w236:bool)
          n116 = Select(t=State."Read Real Data" ("Enum"), s=w236, f=State."Read Simulated Data" ("Enum")) -> (s? t:f=w235:T2)
        }
      }
      n117 = local read "Refresh Rate [s]"() -> (w38:i32)
      n118 = Multiply(x=w38, y=1000) -> (x*y=w41:i32)
      n119 = Divide(x=w41, y=4.0) -> (x/y=w39:dbl)
      n120 = To Long Integer(number=w39) -> (32bit integer=w36:i32)
      n121 = Not Equal?(x=w36, y=w28) -> (x != y?=w43:bool)
      n122 = Or(x=w43, y="stop") -> (x .or. y?=w44:bool)
      n123 = Unbundle By Name(w30) -> ("Waveform"=→"Real-time data":waveform(dbl))
      n124 = node-c288() -> ()  [unwired: 1 in, 1 out]
    }
    n125 = node-c288(w16) -> ()  [unwired: 1 out]
  }
  n126 = call <vilib>:"Butterworth Coefficients.vi"() -> ()  [unwired: 10 in, 2 out]
  n127 = call <vilib>:"Transfer Function PtByPt.vi"() -> ()  [unwired: 5 in, 4 out]
